vi "AutonControl.vi"(7 "Disabled":bool=TRUE, 8 "error in":errorcluster, 9 "Gamepad Data":T1, 10 "HMI to Control":T2, 11 "SensorInputData":T3) -> (0 "error out":errorcluster, 2 "HMI to Control Out":T2, 3 "SensorInputDataOut":T3)   [LabVIEW 2015]
uses:
  Typedefs/SensorInputData.ctl
  Typedefs/HMI_to_Control.ctl
  Typedefs/GamepadData.ctl
  scriptlib/auto_data.vi
panel:
  out "autontime":i32
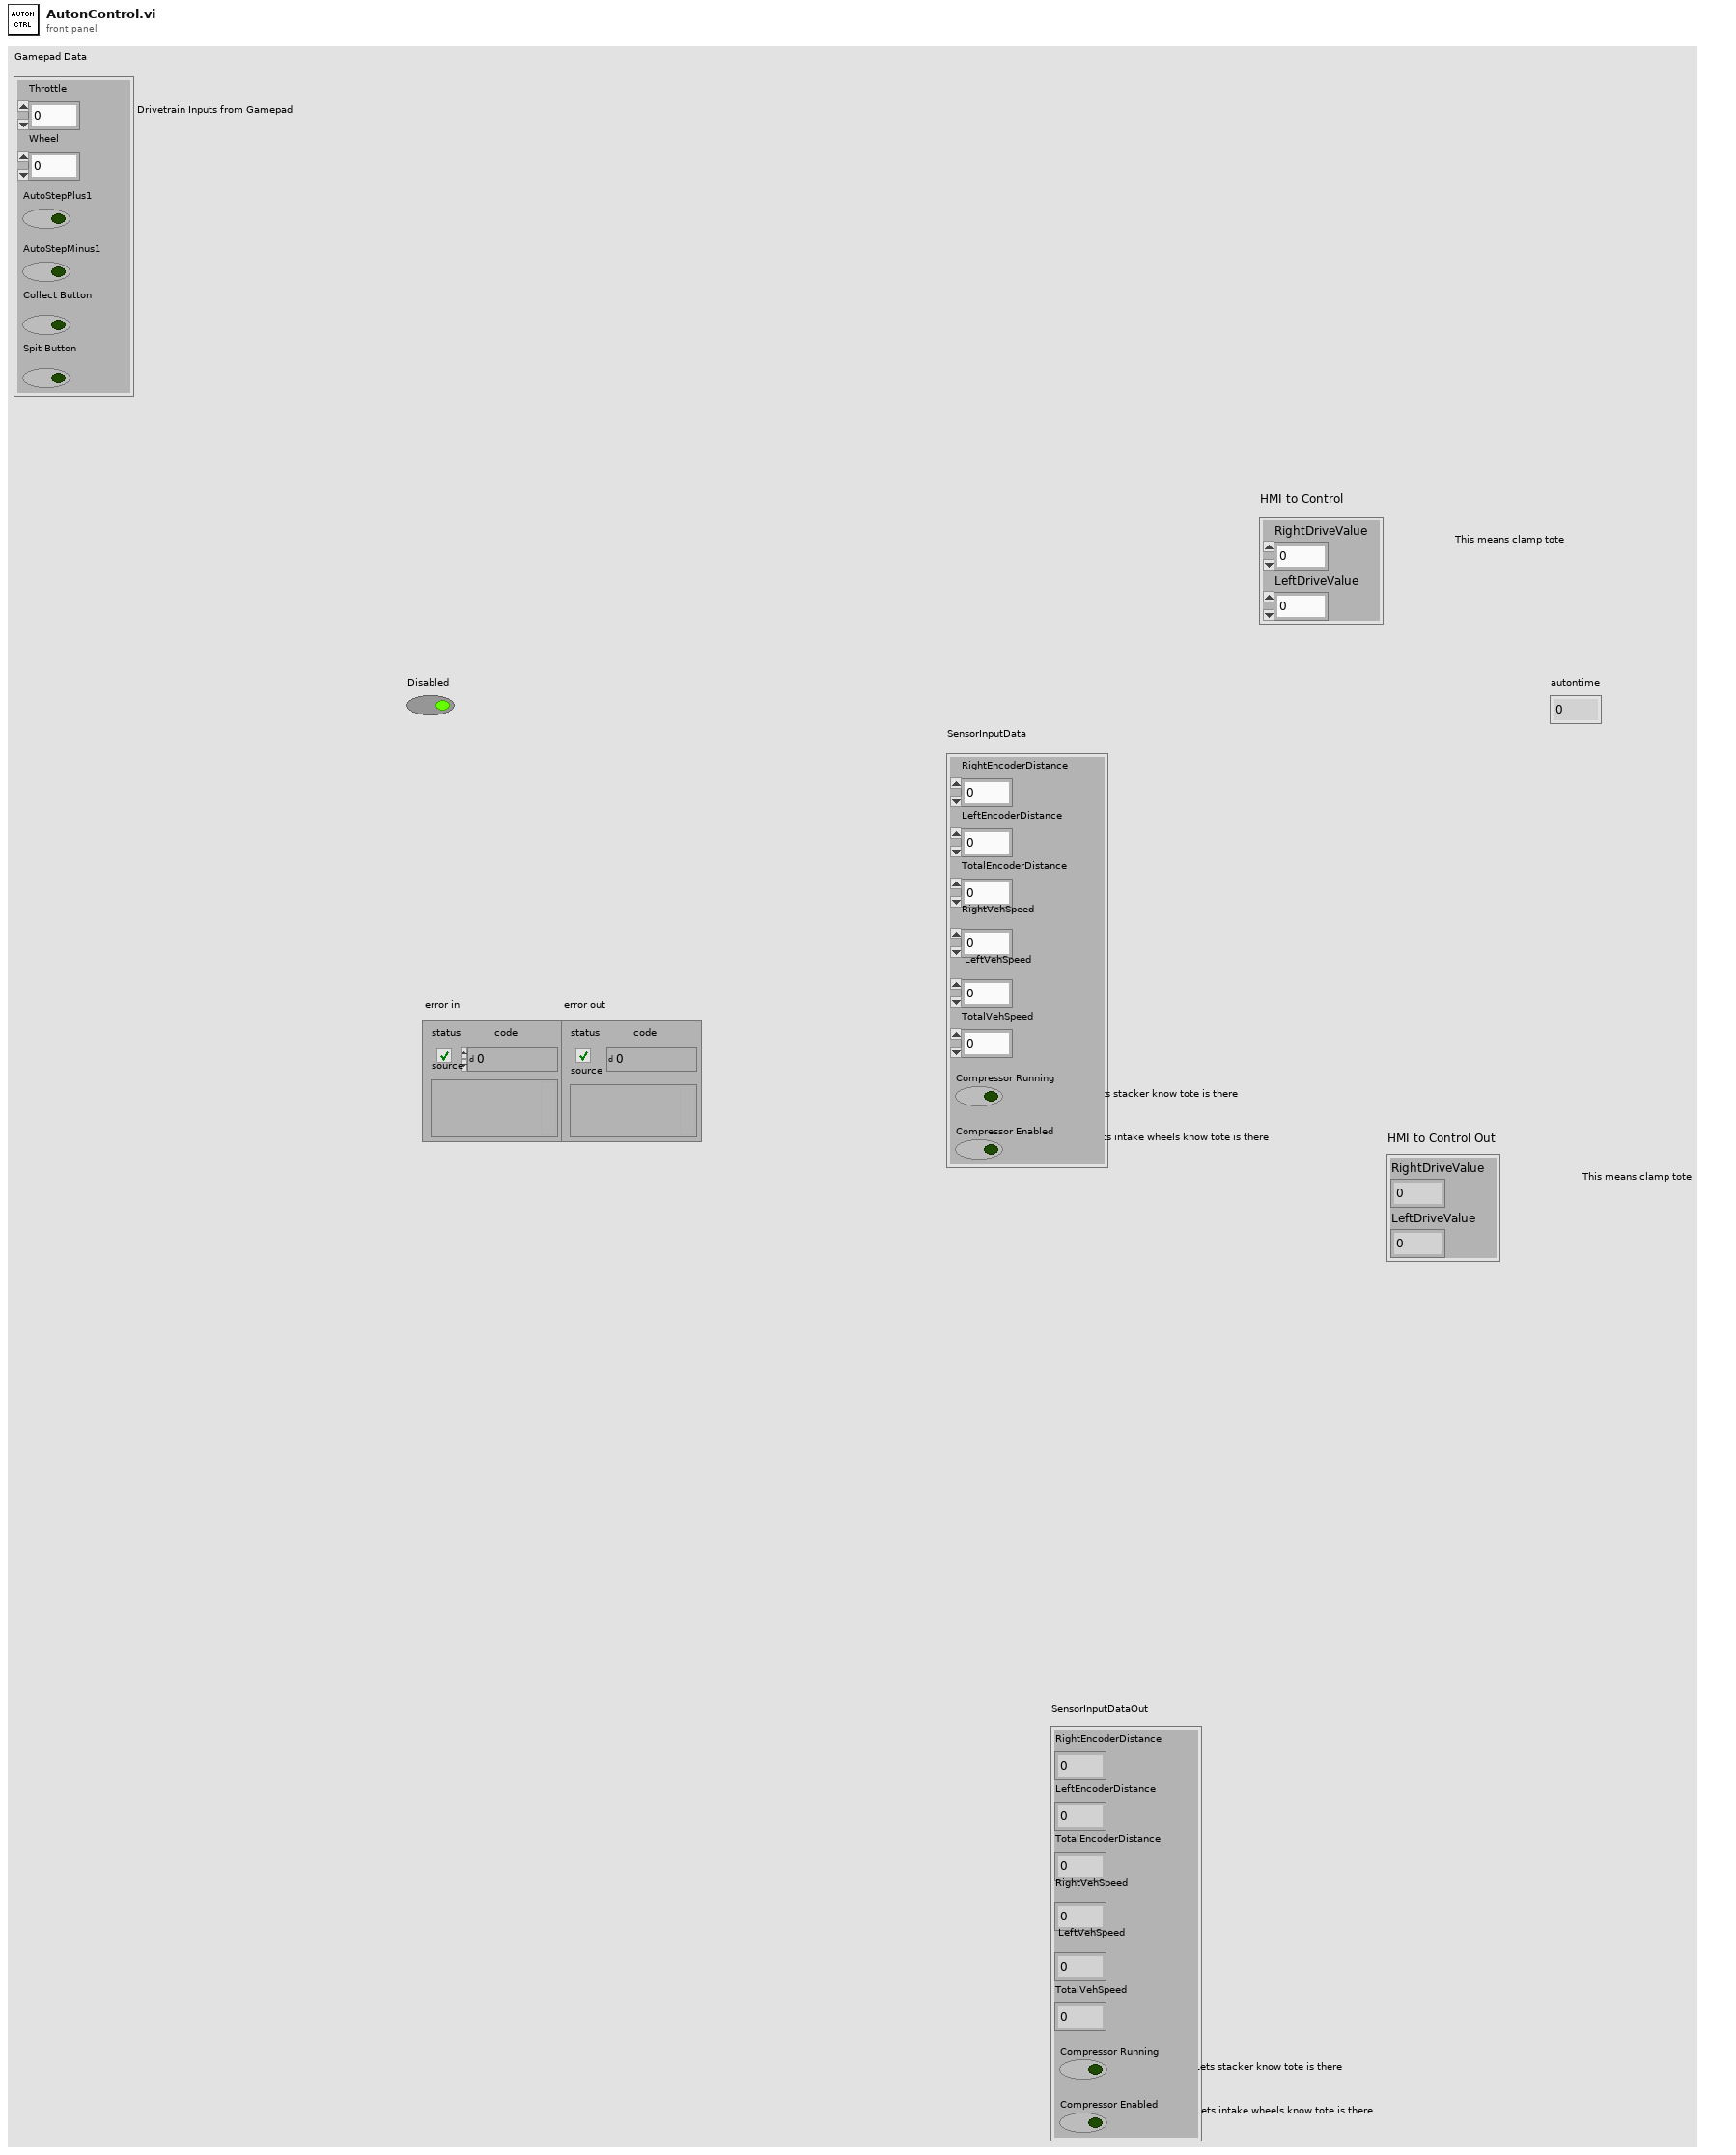
[diagram p1: front panel]
types:
  T1 = typedef "GamepadData.ctl" = cluster{"Throttle":dbl, "Wheel":dbl, "AutoStepPlus1":bool, "AutoStepMinus1":bool, "Collect Button":bool, "Spit Button":bool}
  T2 = typedef "HMI_to_Control.ctl" = cluster{"RightDriveValue":dbl, "LeftDriveValue":dbl}
  T3 = typedef "SensorInputData.ctl" = cluster{"RightEncoderDistance":dbl, "LeftEncoderDistance":dbl, "TotalEncoderDistance":dbl, "RightVehSpeed":dbl, "LeftVehSpeed":dbl, "TotalVehSpeed":dbl, "Compressor Running":bool, "Compressor Enabled":bool}
  T4 = typedef "vi_execute.ctl" = cluster{"arguments":string[], "command":string, "refnum valid check":bool, "vi_ind":u8}
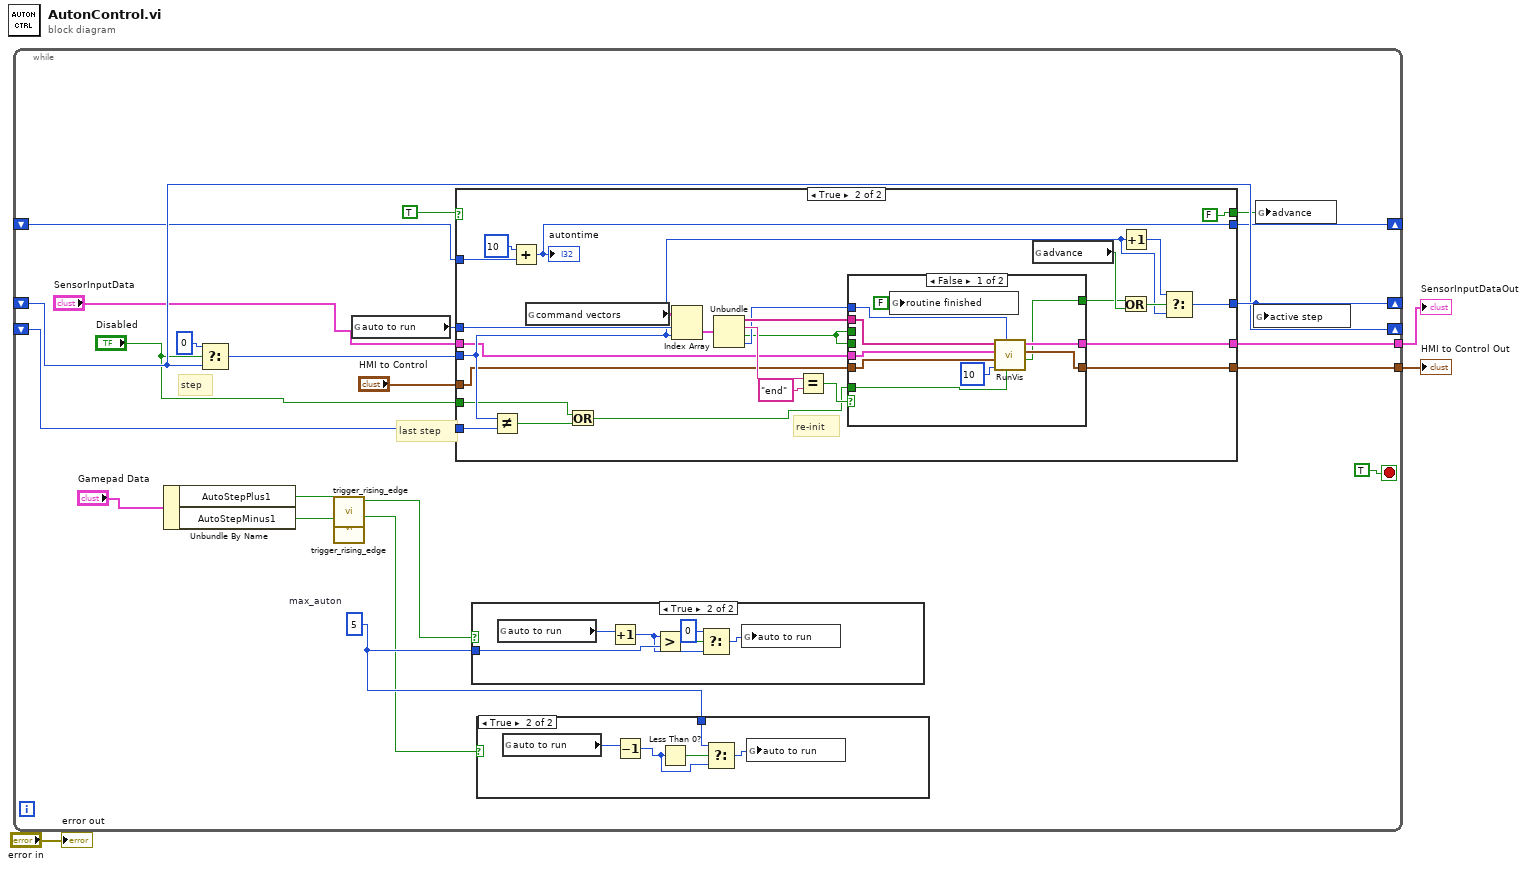
[diagram p0: block diagram]
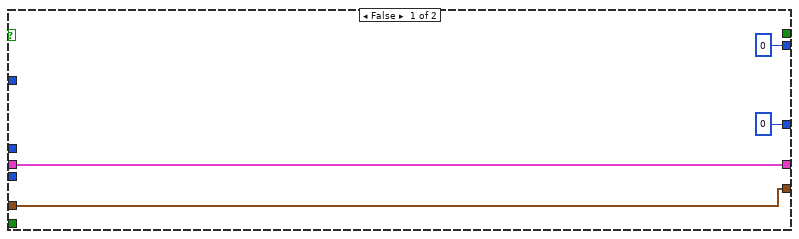
[diagram p4: hidden frame]
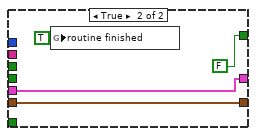
[diagram p5: hidden frame]
diagram:
  n1 = while {
    shift-right: [w22] -> _
    shift-left: _ -> [w21]
    shift-right: [w21] -> _
    shift-left: _ -> [w20]
    shift-right: [w17] -> _
    shift-left: _ -> [w16]
    tunnel: [w14] -> w2
    tunnel: [w13] -> w1
    stop <- TRUE stop-if-true
    w11 = i8 5  # max_auton
    # "last step"
    # "step"
    n2 = Unbundle By Name("Gamepad Data") -> ("AutoStepPlus1"=w10:bool, "AutoStepMinus1"=w8:bool)
    n3 = Select(t=0, s="Disabled", f=w21) -> (s? t:f=w23:i32)
    n4 = call "trigger_rising_edge.vi"("input"=w10) -> ("rising"=w9:bool)  [unwired: 10 in]
    n5 = call "trigger_rising_edge.vi"("input"=w8) -> ("rising"=w7:bool)  [unwired: 10 in]
    n6 = global read "auto_data.vi" "auto to run"() -> (w25:i8)
    n7 = case shown="True" TRUE ("init_done") {
      tunnel: w25 -> [_ w57]
      tunnel: w23 -> [_ w56]
      tunnel: [0 w58] -> w22
      tunnel: w20 -> [_ w55]
      tunnel: [_ FALSE ("advance")] -> w19
      tunnel: [0 w52] -> w17
      tunnel: w16 -> [_ w51]
      tunnel: "SensorInputData" -> [w40 w50]
      tunnel: "HMI to Control" -> [w39 w49]
      tunnel: [w40 w47] -> w14
      tunnel: [w39 w46] -> w13
      tunnel: "Disabled" -> [_ w41]
      frame False {
      }
      frame True {
        # "re-init"
        n8 = Not Equal?(x=w56, y=w55) -> (x != y?=w43:bool)
        n9 = Add(x=10, y=w51) -> (x+y=w52:i32)
        "autontime" <- w52
        n10 = global read "auto_data.vi" "command vectors"() -> (w67:T4[][])
        n11 = Or(x=w41, y=w43) -> (x .or. y?=w42:bool)
        n12 = Index Array(array=w67, index (row)=w57, index (col)=w56) -> (element=w66:T4)
        n13 = Unbundle(w66) -> ("arguments"=w65:string[], "command"=w64:string, "refnum valid check"=w44:bool, "vi_ind"=w48:u8)
        n14 = Equal?(x=w64, y="end") -> (x = y?=w62:bool)
        n15 = case shown="False" w62 {
          tunnel: w65 -> [w74 _]
          tunnel: w50 -> [w76 w79]
          tunnel: w49 -> [w75 w78]
          tunnel: w48 -> [w73 _]
          tunnel: w42 -> [w71 _]
          tunnel: [w70 w79] -> w47
          tunnel: [w69 w78] -> w46
          tunnel: [w68 FALSE ("Done")] -> w45
          tunnel: w44 -> [_ _]
          tunnel: w44 -> [_ _]
          frame False {
            n16 = global write "auto_data.vi" "routine finished"(FALSE ("routine finished")) -> ()
            n17 = call "RunVis.vi"("Re-Init"=w71, "Index"=w73, "dt"=i8 10, "HMI to Control"=w75, "SensorInputData"=w76, "arguments"=w74) -> ("Done"=w68:bool, "HMI to Control Out"=w69:T2, "SensorInputDataOut"=w70:T3)  [unwired: 3 in]
          }
          frame True {
            n18 = global write "auto_data.vi" "routine finished"(TRUE ("routine finished")) -> ()
          }
        }
        n19 = global read "auto_data.vi" "advance"() -> (w61:bool)
        n20 = Increment(x=w56) -> (x+1=w59:i32)
        n21 = Or(x=w45, y=w61) -> (x .or. y?=w60:bool)
        n22 = Select(t=w59, s=w60, f=w56) -> (s? t:f=w58:i32)
      }
    }
    n23 = case shown="True" w9 {
      tunnel: w11 -> [_ w34]
      frame False {
      }
      frame True {
        n24 = global read "auto_data.vi" "auto to run"() -> (w36:i8)
        n25 = Increment(x=w36) -> (x+1=w33:i8)
        n26 = Greater?(x=w33, y=w34) -> (0:w35:bool)
        n27 = Select(t=i8 0, s=w35, f=w33) -> (s? t:f=w31:i8)
        n28 = global write "auto_data.vi" "auto to run"(w31) -> ()
      }
    }
    n29 = case shown="True" w7 {
      tunnel: w11 -> [_ w27]
      frame False {
      }
      frame True {
        n30 = global read "auto_data.vi" "auto to run"() -> (w30:i8)
        n31 = Decrement(x=w30) -> (x-1=w26:i8)
        n32 = Less Than 0?(x=w26) -> (x < 0?=w29:bool)
        n33 = Select(t=w27, s=w29, f=w26) -> (s? t:f=w28:i8)
        n34 = global write "auto_data.vi" "auto to run"(w28) -> ()
      }
    }
    n35 = global write "auto_data.vi" "active step"(w22) -> ()
    n36 = global write "auto_data.vi" "advance"(w19) -> ()
  }
  "SensorInputDataOut" <- w2
  "HMI to Control Out" <- w1
  "error out" <- "error in"
